vi "Send command ADC.vi"(8 "error in (no error)":errorcluster, 9 "Canal":string(combo), 10 "Marca":string, 11 "object in":refnum<class "NXP.lvclass">) -> (0 "error out":errorcluster, 1 "Expected response":string, 2 "Command":string, 3 "object out":refnum<class "NXP.lvclass">)   [LabVIEW 2020, in "NXP.lvclass"]
doc: "Se manda el comando para leer el ADC, se escribe en el puerto serial y se lee la respuesta que de el micro."
uses:
  NXP.lvclass
  NXP.lvclass/NXP.ctl
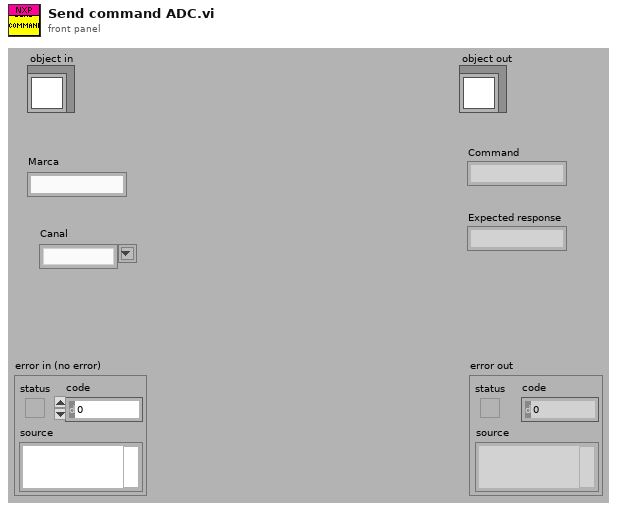
[diagram p1: front panel]
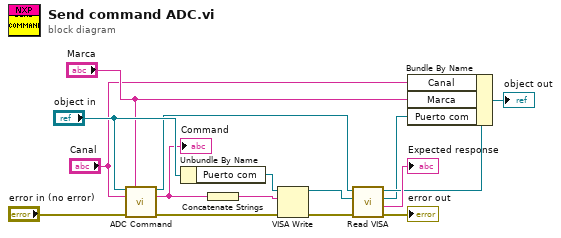
[diagram p0: block diagram]
diagram:
  n1 = call-dynamic "ADC Command.vi"("object in"="object in", "Marca"="Marca", "Canal"="Canal", "error in (no error)"="error in (no error)") -> ("object out"=w4:refnum<class "NXP.lvclass">, "Command"=w9:string, "error out"=w11:errorcluster)  [unwired: 8 in, 1 out]
  "Command" <- w9
  n2 = Unbundle By Name("object in") -> ("Puerto com"=w15:refnum<visa-resource-name>)
  n3 = Concatenate Strings(w9) -> (w16:string)
  n4 = VISA Write(VISA resource name=w15, write buffer=w16, error in (no error)=w11) -> (VISA resource name out=w8:refnum<visa-resource-name>, error out=w7:errorcluster)  [unwired: 1 out]
  n5 = call-dynamic "Read VISA.vi"("error in (no error)"=w7, "VISA Refnum in"=w8, "Serial Device in"=w4) -> ("error out"=→"error out":errorcluster, "Serial Response"=→"Expected response":string, "VISA resource name out"=w2:refnum<visa-resource-name>, "Serial Device out"=w3:refnum<class "NXP.lvclass">)  [unwired: 5 in]
  n6 = Bundle By Name(cluster=w3, "Canal"="Canal", "Marca"="Marca", "Puerto com"=w2) -> (→"object out":refnum<class "NXP.lvclass">)
